vi "init.vi"(8 "error in (no error)":errorcluster, 11 "FlukeDMMTC in":refnum<class "FlukeDMMTC.lvclass">) -> (0 "error out":errorcluster, 3 "FlukeDMMTC out":refnum<class "FlukeDMMTC.lvclass">)   [LabVIEW 2013, in "FlukeDMMTC.lvclass"]
uses:
  FlukeDMMTC.lvclass
  <userlib>/Common/Devices/FlukeDMM/Config/FlukeDMM.ctl
  <userlib>/Common/SerialProtocols/Configuration/SerialConfig.ctl
  <userlib>/Common/SerialProtocols/Configuration/SerialProtocol.ctl
  <userlib>/Common/SerialProtocols/Configuration/ProtocolParameters.ctl
  <userlib>/Common/SerialProtocols/Configuration/SerialMessageParameters.ctl
  <userlib>/Common/Devices/FlukeDMM/FlukeDMM/FlukeDMM.lvclass/FlukeDMM.ctl
  <userlib>/Common/Devices/FlukeDMM/FlukeDMM/FlukeDMM.lvclass
  ConfigurationThisComponent/ConfigurationThisComponent.lvclass
  <userlib>/Common/SerialProtocols/SerialProtocols.lvlib
  <userlib>/Common/Devices/FlukeDMM/FlukeDMM.lvlib
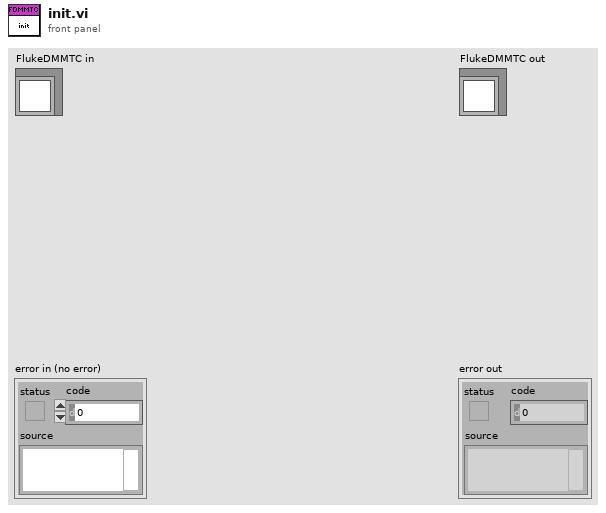
[diagram p1: front panel]
types:
  T1 = typedef "FlukeDMM.lvlib/FlukeDMM.ctl" = cluster{"Serial":T2}
  T2 = typedef "SerialProtocols.lvlib/SerialConfig.ctl" = cluster{"Serial Protocol":T3, "Protocol Parameters":T4, "Serial Message Parameters":T5}
  T3 = typedef "SerialProtocols.lvlib/SerialProtocol.ctl" = enum16{"RS232", "RS485", "SerialSimulator"}
  T4 = typedef "SerialProtocols.lvlib/ProtocolParameters.ctl" = cluster{"VISA resource name":refnum<visa-resource-name>, "Baud Rate":u32, "Data Bits":u16, "Parity":enum16{"None", "Odd", "Even", "Mark", "Space"}, "Flow Control":u16, "Stop Bits":u16, "Timeout (ms)":u32}
  T5 = typedef "SerialProtocols.lvlib/SerialMessageParameters.ctl" = cluster{"Byte Count":u32, "Enable Termination Character":bool, "Termination Char":u8}
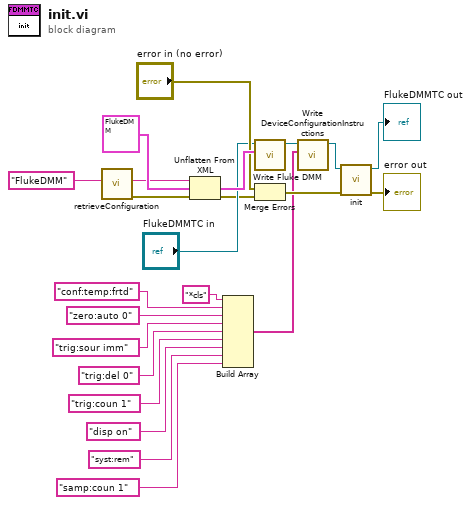
[diagram p0: block diagram]
diagram:
  n1 = call "retrieveConfiguration.vi"("configName"="FlukeDMM") -> ("error out"=w17:errorcluster, "xmlConfig"=w19:string)  [unwired: 8 in, 1 out]
  n2 = Unflatten From XML(xml string=w19, type=T1 {"Serial"={"Serial Protocol"=enum."RS485", "Protocol Parameters"={"VISA resource name"="", "Baud Rate"=9600, "Data Bits"=8, "Parity"=enum."None", "Flow Control"=0, "Stop Bits"=10, "Timeout (ms)"=10000}, "Serial Message Parameters"={"Byte Count"=200, "Enable Termination Character"=FALSE, "Termination Char"=200}}} ("Fluke DMM"), error in (no error)=w17) -> (value=w18:T1, error out=w1:errorcluster)
  n3 = Build Array("*cls" ("writeString"), "conf:temp:frtd" ("writeString"), "zero:auto 0" ("writeString"), "trig:sour imm" ("writeString"), "trig:del 0" ("writeString"), "trig:coun 1" ("writeString"), "disp on" ("writeString"), "syst:rem" ("writeString"), "samp:coun 1" ("writeString")) -> (w5:string[])
  n4 = call <userlib>:"Write Fluke DMM.vi"("Fluke DMM"=w18, "FlukeDMM in"="FlukeDMMTC in") -> ("FlukeDMM out"=w3:refnum<class "FlukeDMMTC.lvclass">)  [unwired: 9 in]
  n5 = Merge Errors("error in (no error)", w1) -> (w15:errorcluster)
  n6 = call <userlib>:"Write DeviceConfigurationInstructions.vi"("DeviceConfigurationInstructions"=w5, "FlukeDMM in"=w3) -> ("FlukeDMM out"=w2:refnum<class "FlukeDMMTC.lvclass">)  [unwired: 9 in]
  n7 = call-parent "init.vi"("error in (no error)"=w15, "FlukeDMM in"=w2) -> ("error out"=→"error out":errorcluster, "FlukeDMM out"=→"FlukeDMMTC out":refnum<class "FlukeDMMTC.lvclass">)  [unwired: 8 in]
